vi "IsLogFileSizeTriggered.vi"(8 "Error In":errorcluster, 11 "File Size (MB)":u32) -> (0 "Error Out":errorcluster, 3 "Triggered?":bool)   [LabVIEW 2013]
uses:
  LogFileGlobalAction.ctl
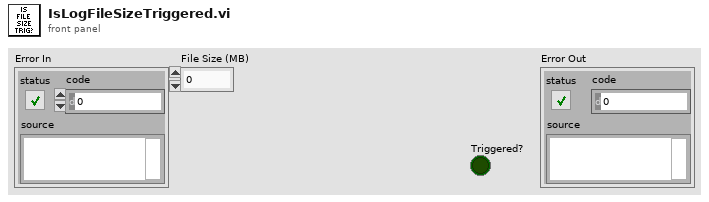
[diagram p1: front panel]
types:
  T1 = typedef "LogFileGlobalAction.ctl" = enum16{"Open", "Write", "Size", "Close"}
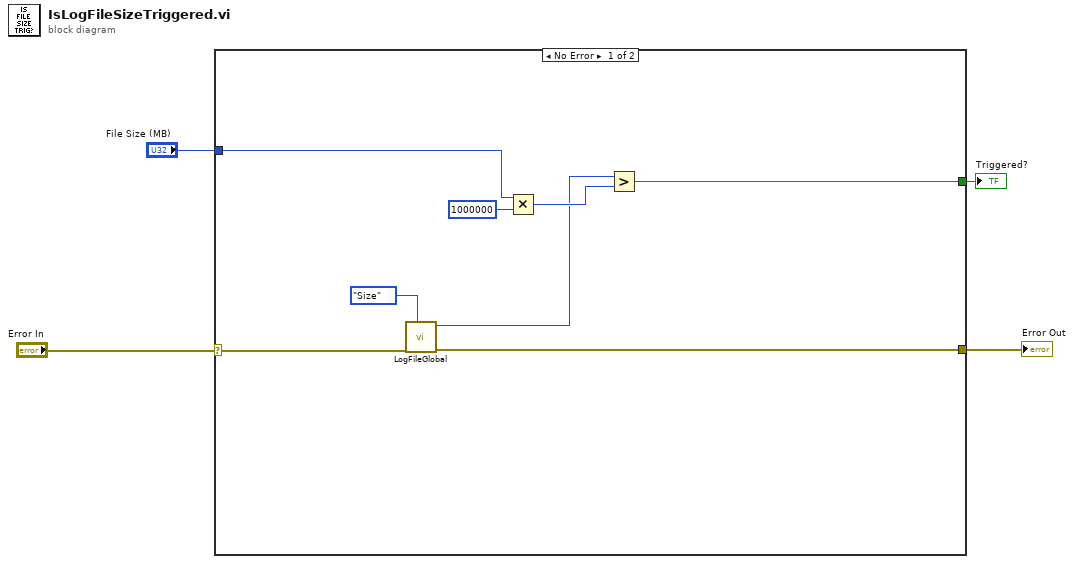
[diagram p0: block diagram]
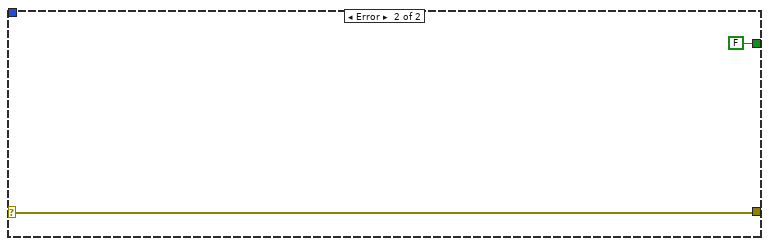
[diagram p2: hidden frame]
diagram:
  n1 = case shown="No Error" "Error In" {
    selector: "Error In" -> [w5 w13]
    tunnel: [w6 w13] -> w3
    tunnel: "File Size (MB)" -> [w10 _]
    tunnel: [w9 FALSE] -> w1
    frame No Error {
      n2 = call "LogFileGlobal.vi"("Action"=LogFileGlobalAction."Size", "Error In"=w5) -> ("Error Out"=w6:errorcluster, "Size (bytes)"=w7:i64)  [unwired: 8 in]
      n3 = Multiply(x=w10, y=u32 1000000) -> (x*y=w11:u32)
      n4 = Greater?(x=w7, y=w11) -> (0:w9:bool)
    }
    frame Error {
    }
  }
  "Error Out" <- w3
  "Triggered?" <- w1
